vi "Limelight Published Globals.vi"() -> ()   [LabVIEW 2018]
doc: "This is used primarily to publish values that other subsystems or user code may want to read periodically. It may also contain some settings such as debug switches or implementation selections that are independent of the operating mode of the subsystem."
uses:
  Limelight Setpoints.ctl
  Limelight Operations.ctl
  <vilib>/Rock Robotics/WPI/Framework/Command Status Info.ctl
  <vilib>/Rock Robotics/WPI/Framework/Completion Status.ctl
  <vilib>/Rock Robotics/WPI/Framework/Completion Notifier.ctl
  Pipeline Index.ctl
panel:
  out "Skew/Rotation":dbl
  out "Target Area":dbl
  out "Vertical Offset":dbl
  out "Horizontal Offset":dbl
  out "Pipeline":T1
  out "Target Found?":bool
  in  "Current Command":T7
  # "Tip: The global is a good way publish state or\ninformational/debugging values.\nIt is not  advised that you put setpoint values here."
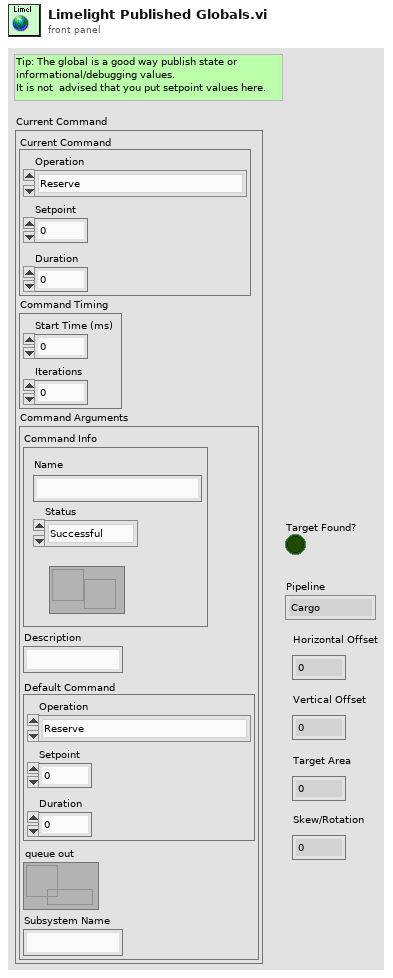
[diagram p1: front panel]
types:
  T1 = typedef "Pipeline Index.ctl" = enum16{"Cargo", "Hatch", "Vision"}
  T2 = typedef "Limelight Setpoints.ctl" = cluster{"Operation":T3, "Setpoint":dbl, "Duration":dbl}
  T3 = typedef "Limelight Operations.ctl" = enum16{"Reserve", "Read Current", "Immediate", "Pipeline Change"}
  T4 = typedef "Command Status Info.ctl" = cluster{"Name":string, "Status":T5, "notifier out":T6}
  T5 = typedef "Completion Status.ctl" = enum16{"Successful", "Aborted", "Incomplete"}
  T6 = typedef "Completion Notifier.ctl" = refnum<notifier>
  T7 = cluster{"Current Command":T2, "Command Timing":cluster{"Start Time (ms)":u32, "Iterations":i32}, "Command Arguments":cluster{"Command Info":T4, "Description":string, "Default Command":T2, "queue out":refnum<queue>, "Subsystem Name":string}}
diagram:
